vi "MyPAM FPGA Safety Block.vi"() -> ()   [LabVIEW 2015]
panel:
  in  "MOTOR2_DEM_CURR":i16
  in  "MOTOR1_DEM_CURR":i16
  out "SAFETY":T1
  in  "MOTOR1_DEM_CURR_MAX_CHANGE":i16
  in  "MOTOR2_DEM_CURR_MAX_CHANGE":i16
  in  "MOTOR2_PWM_MAX":i16
  in  "MOTOR1_PWM_MAX":i16
  in  "MOTOR2_PWM":i16
  in  "MOTOR1_PWM":i16
  in  "EEPOS_Y_MIN_MM":fxp<+/-,32,24>
  in  "EEPOS_Y_MAX_MM":fxp<+/-,32,24>
  in  "EEPOS_X_MM":fxp<+/-,32,24>
  in  "EEPOS_Y_MM":fxp<+/-,32,24>
  in  "EEPOS_X_MIN_MM":fxp<+/-,32,24>
  in  "EEPOS_X_MAX_MM":fxp<+/-,32,24>
  in  "ALLOWED_DEG_ERROR":fxp<+/-,32,24>
  in  "POT_2_DEG":fxp<+/-,32,24>
  in  "POT_1_DEG":fxp<+/-,32,24>
  in  "ENC_2_DEG":fxp<+/-,32,24>
  in  "ENC_1_DEG":fxp<+/-,32,24>
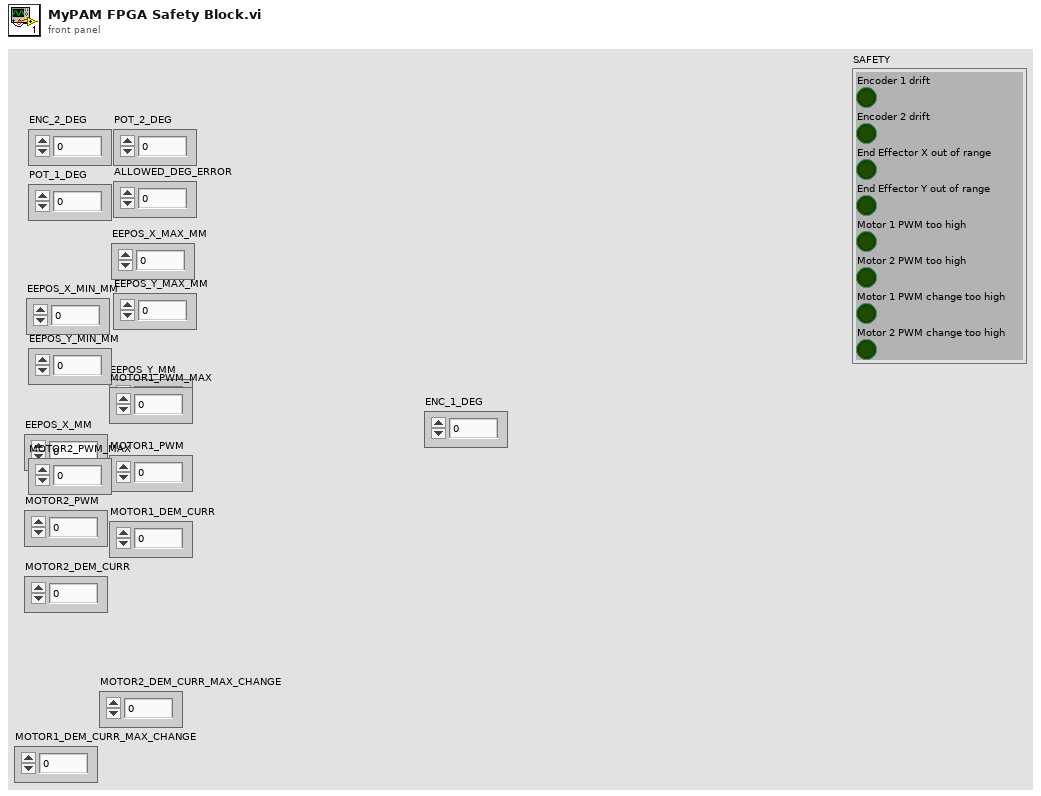
[diagram p1: front panel]
types:
  T1 = cluster{"Encoder 1 drift":bool, "Encoder 2 drift":bool, "End Effector X out of range":bool, "End Effector Y out of range":bool, "Motor 1 PWM too high":bool, "Motor 2 PWM too high":bool, "Motor 1 PWM change too high":bool, "Motor 2 PWM change too high":bool}
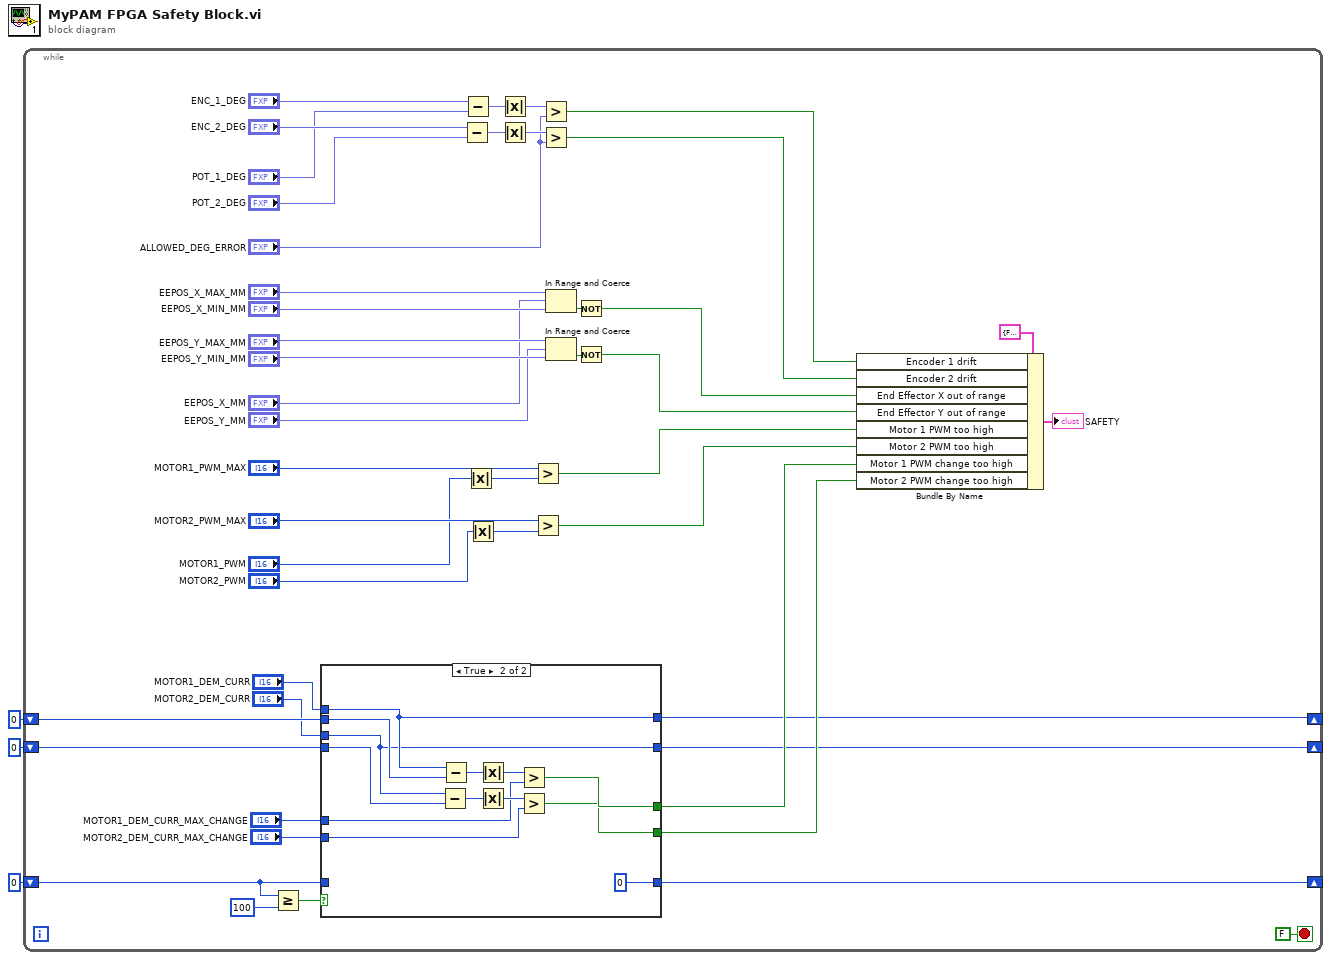
[diagram p0: block diagram]
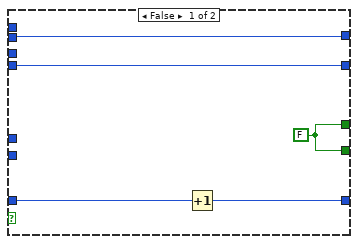
[diagram p2: hidden frame]
diagram:
  n1 = while {
    shift-right: [w10] -> _
    shift-left: i16 0 ("MOTOR1_PWM") -> [w20]
    shift-right: [w9] -> _
    shift-left: i16 0 ("MOTOR1_PWM") -> [w19]
    shift-right: [w13] -> _
    shift-left: u8 0 ("MOTOR1_PWM") -> [w6]
    stop <- FALSE stop-if-true
    n2 = Greater Or Equal?(x=w6, y=u8 100 ("MOTOR1_PWM")) -> (x >= y?=w8:bool)
    n3 = case shown="True" w8 {
      tunnel: "MOTOR1_DEM_CURR" -> [_ w56]
      tunnel: w20 -> [w52 w63]
      tunnel: w19 -> [w51 w62]
      tunnel: "MOTOR2_DEM_CURR" -> [_ w55]
      tunnel: "MOTOR1_DEM_CURR_MAX_CHANGE" -> [_ w61]
      tunnel: "MOTOR2_DEM_CURR_MAX_CHANGE" -> [_ w60]
      tunnel: [w53 w59] -> w15
      tunnel: [w53 w58] -> w14
      tunnel: [w54 u8 0 ("MOTOR1_PWM")] -> w13
      tunnel: [w52 w56] -> w10
      tunnel: [w51 w55] -> w9
      tunnel: w6 -> [w50 _]
      frame False {
        w53 = FALSE
        n4 = Increment(x=w50) -> (x+1=w54:u8)
      }
      frame True {
        n5 = Subtract(x=w55, y=w62) -> (x-y=w64:i16)
        n6 = Subtract(x=w56, y=w63) -> (x-y=w65:i16)
        n7 = Absolute Value(x=w65) -> (abs(x)=w66:i16)
        n8 = Absolute Value(x=w64) -> (abs(x)=w67:i16)
        n9 = Greater?(x=w66, y=w61) -> (0:w59:bool)
        n10 = Greater?(x=w67, y=w60) -> (0:w58:bool)
      }
    }
    n11 = Subtract(x="ENC_2_DEG", y="POT_2_DEG") -> (x-y=w45:fxp<+/-,33,25>)
    n12 = Subtract(x="ENC_1_DEG", y="POT_1_DEG") -> (x-y=w44:fxp<+/-,33,25>)
    n13 = Absolute Value(x="MOTOR1_PWM") -> (abs(x)=w32:i16)
    n14 = Absolute Value(x="MOTOR2_PWM") -> (abs(x)=w30:i16)
    n15 = Absolute Value(x=w44) -> (abs(x)=w43:fxp<+,32,24>)
    n16 = Absolute Value(x=w45) -> (abs(x)=w42:fxp<+,32,24>)
    n17 = Greater?(x="MOTOR1_PWM_MAX", y=w32) -> (0:w23:bool)
    n18 = Greater?(x="MOTOR2_PWM_MAX", y=w30) -> (0:w22:bool)
    n19 = Greater?(x=w43, y="ALLOWED_DEG_ERROR") -> (0:w27:bool)
    n20 = Greater?(x=w42, y="ALLOWED_DEG_ERROR") -> (0:w26:bool)
    n21 = In Range and Coerce(upper limit="EEPOS_X_MAX_MM", x="EEPOS_X_MM", lower limit="EEPOS_X_MIN_MM") -> (In Range?=w34:bool)  [unwired: 1 out]
    n22 = In Range and Coerce(upper limit="EEPOS_Y_MAX_MM", x="EEPOS_Y_MM", lower limit="EEPOS_Y_MIN_MM") -> (In Range?=w33:bool)  [unwired: 1 out]
    n23 = Not(x=w34) -> (.not. x?=w25:bool)
    n24 = Not(x=w33) -> (.not. x?=w24:bool)
    n25 = Bundle By Name(cluster=T1 {"Encoder 1 drift"=FALSE, "Encoder 2 drift"=FALSE, "End Effector X out of range"=FALSE, "End Effector Y out of range"=FALSE, "Motor 1 PWM too high"=FALSE, "Motor 2 PWM too high"=FALSE, "Motor 1 PWM change too high"=FALSE, "Motor 2 PWM change too high"=FALSE} ("SAFETY"), "Encoder 1 drift"=w27, "Encoder 2 drift"=w26, "End Effector X out of range"=w25, "End Effector Y out of range"=w24, "Motor 1 PWM too high"=w23, "Motor 2 PWM too high"=w22, "Motor 1 PWM change too high"=w15, "Motor 2 PWM change too high"=w14) -> (→"SAFETY":T1)
  }
